vi "Data Transmission DAO.vi"(7 "refnum":T1, 8 "error in (no error)":errorcluster, 9 "Port Number In":u16, 10 "Wait For Notification Timeout In":i32=1000, 11 "Persistent DAO Actions":T2) -> (0 "error out":errorcluster, 1 "Port Number Out":u16, 2 "Wait For Notification Timeout Out":i32=1000, 3 "Notification Name Out":string="DataAvailableForTransmission", 4 "refnum out":T1)   [LabVIEW 2009]
uses:
  Metadata/Persistant DAO Actions.ctl
  <vilib>/Utility/config.llb/Config Data RefNum.ctl
  <vilib>/Utility/config.llb/Read Key (String).vi
  <vilib>/Utility/config.llb/Read Key (I32).vi
  <vilib>/Utility/config.llb/Read Key (U32).vi
  <vilib>/Utility/config.llb/Write Key (String).vi
  <vilib>/Utility/config.llb/Write Key (I32).vi
  <vilib>/Utility/config.llb/Write Key (U32).vi
  <vilib>/Utility/config.llb/NI_LVConfig.lvlib
panel:
  in  "Notification Name In":string="DataAvailableForTransmission"
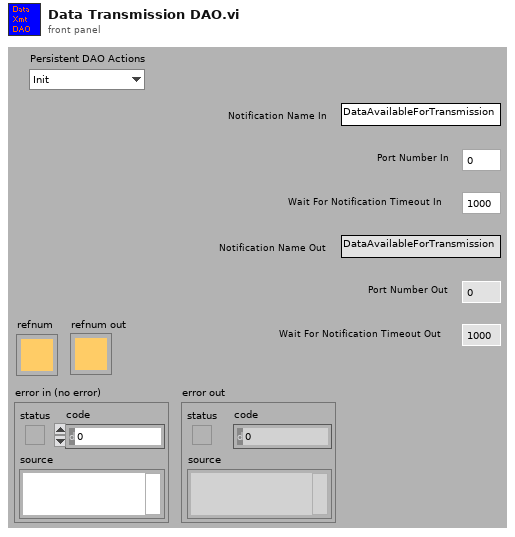
[diagram p1: front panel]
types:
  T1 = typedef "NI_LVConfig.lvlib/Config Data RefNum.ctl" = refnum<k1>
  T2 = typedef "Persistant DAO Actions.ctl" = enum16{"Init", "Get", "Set", "Load", "Save"}
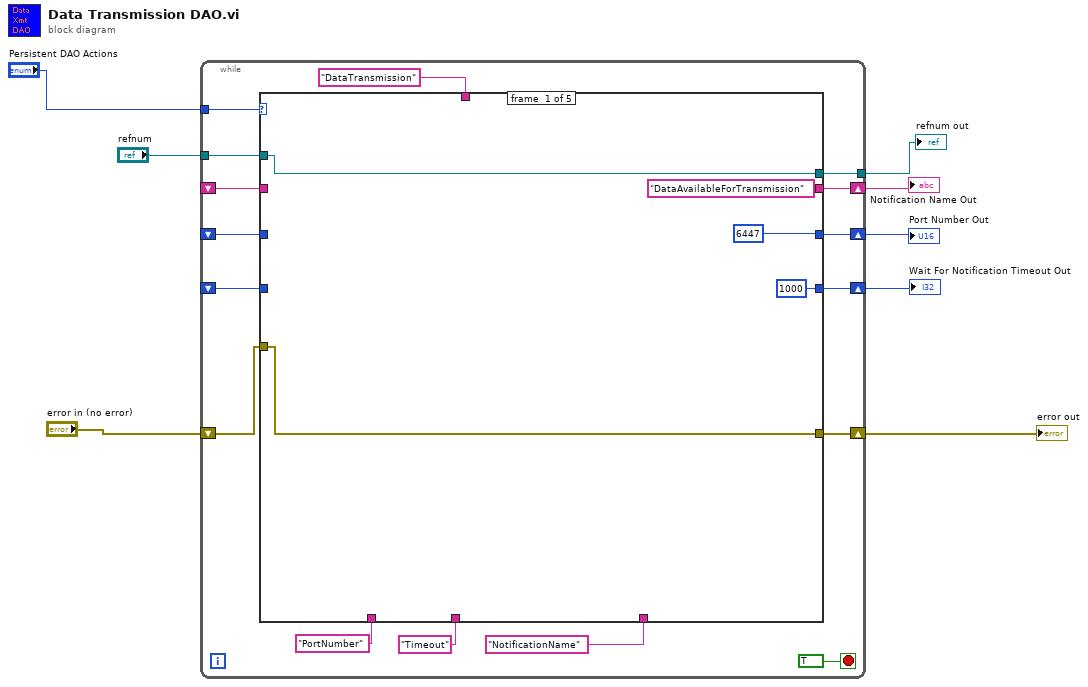
[diagram p0: block diagram]
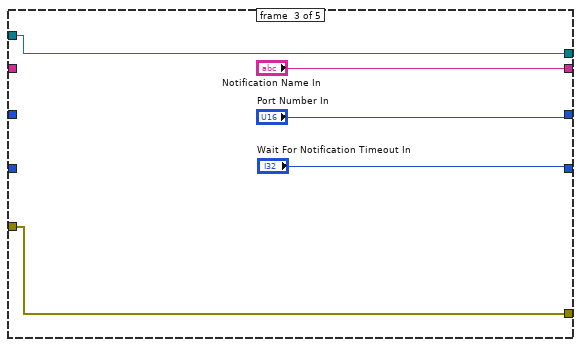
[diagram p3: hidden frame]
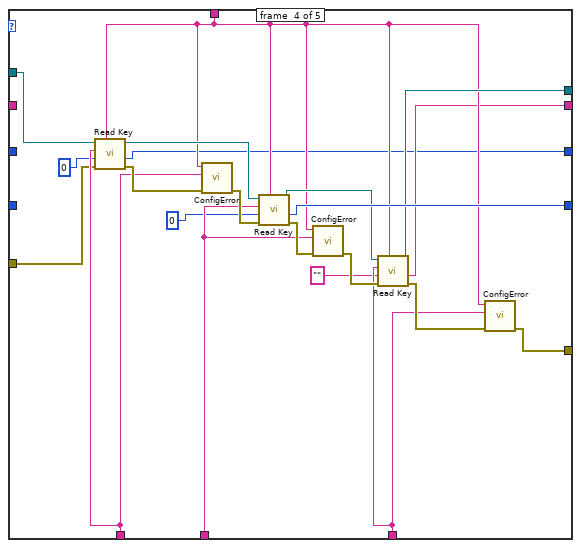
[diagram p4: hidden frame]
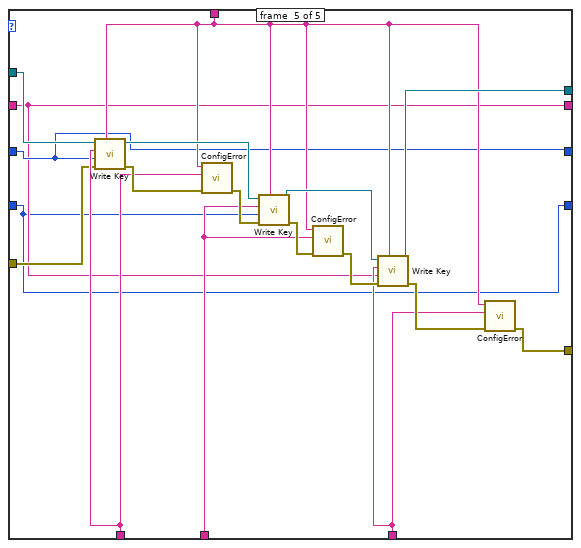
[diagram p5: hidden frame]
diagram:
  n1 = while {
    tunnel: "Persistent DAO Actions" -> [w23]
    shift-right: [w22] -> w7
    shift-left: _ -> [w20]
    shift-right: [w21] -> w6
    shift-left: _ -> [w19]
    shift-right: [w18] -> w5
    shift-left: _ -> [w17]
    tunnel: "refnum" -> [w14]
    shift-right: [w11] -> w2
    shift-left: "error in (no error)" -> [w12]
    tunnel: [w10] -> w1
    stop <- TRUE stop-if-true
    n2 = case shown="\"Save\"" w23 {
      tunnel: ["DataAvailableForTransmission" ("Notification Name In") w34 "Notification Name In" w43 w62] -> w22
      tunnel: [u16 6447 ("Port Number In") w30 "Port Number In" w41 w63] -> w21
      tunnel: w20 -> [_ w34 _ _ w62]
      tunnel: w19 -> [_ w30 _ _ w63]
      tunnel: [1000 ("Wait For Notification Timeout In") w33 "Wait For Notification Timeout In" w52 w61] -> w18
      tunnel: w17 -> [_ w33 _ _ w61]
      tunnel: "DataTransmission" -> [_ _ _ w46 w66]
      tunnel: "PortNumber" -> [_ _ _ w59 w77]
      tunnel: w14 -> [w27 w31 w36 w58 w76]
      tunnel: "Timeout" -> [_ _ _ w54 w72]
      tunnel: w12 -> [w26 w32 w37 w51 w71]
      tunnel: [w26 w32 w37 w42 w64] -> w11
      tunnel: [w27 w31 w36 w47 w67] -> w10
      tunnel: "NotificationName" -> [_ _ _ w45 w65]
      frame #0 {
      }
      frame #1 {
      }
      frame #2 {
      }
      frame #3 {
        n3 = call-poly <vilib>:"Read Key.vi"("section"=w46, "error in (no error)"=w51, "default value"=u16 0 ("Port Number In"), "key"=w59, "refnum"=w58) -> ("error out"=w60:errorcluster, "value"=w41:u32, "refnum out"=w55:T1)  [unwired: 4 out]
        n4 = call "ConfigError.vi"("error in (no error)"=w60, "Key"=w59, "Section"=w46) -> ("error out"=w56:errorcluster)  [unwired: 8 out]
        n5 = call-poly <vilib>:"Read Key.vi"("section"=w46, "error in (no error)"=w56, "default value"=0 ("Wait For Notification Timeout In"), "key"=w54, "refnum"=w55) -> ("error out"=w57:errorcluster, "value"=w52:i32, "refnum out"=w48:T1)  [unwired: 4 out]
        n6 = call "ConfigError.vi"("error in (no error)"=w57, "Key"=w54, "Section"=w46) -> ("error out"=w49:errorcluster)  [unwired: 8 out]
        n7 = call-poly <vilib>:"Read Key.vi"("section"=w46, "error in (no error)"=w49, "default value"="", "key"=w45, "refnum"=w48) -> ("error out"=w50:errorcluster, "value"=w43:string, "refnum out"=w47:T1)  [unwired: 1 in, 3 out]
        n8 = call "ConfigError.vi"("error in (no error)"=w50, "Key"=w45, "Section"=w46) -> ("error out"=w42:errorcluster)  [unwired: 8 out]
      }
      frame #4 {
        n9 = call-poly <vilib>:"Write Key.vi"("section"=w66, "error in (no error)"=w71, "value"=w63, "key"=w77, "refnum"=w76) -> ("error out"=w78:errorcluster, "refnum out"=w73:T1)  [unwired: 5 out]
        n10 = call "ConfigError.vi"("error in (no error)"=w78, "Key"=w77, "Section"=w66) -> ("error out"=w74:errorcluster)  [unwired: 8 out]
        n11 = call-poly <vilib>:"Write Key.vi"("section"=w66, "error in (no error)"=w74, "value"=w61, "key"=w72, "refnum"=w73) -> ("error out"=w75:errorcluster, "refnum out"=w68:T1)  [unwired: 5 out]
        n12 = call "ConfigError.vi"("error in (no error)"=w75, "Key"=w72, "Section"=w66) -> ("error out"=w69:errorcluster)  [unwired: 8 out]
        n13 = call-poly <vilib>:"Write Key.vi"("section"=w66, "error in (no error)"=w69, "value"=w62, "key"=w65, "refnum"=w68) -> ("error out"=w70:errorcluster, "refnum out"=w67:T1)  [unwired: 1 in, 4 out]
        n14 = call "ConfigError.vi"("error in (no error)"=w70, "Key"=w65, "Section"=w66) -> ("error out"=w64:errorcluster)  [unwired: 8 out]
      }
    }
  }
  "Port Number Out" <- w6
  "Notification Name Out" <- w7
  "error out" <- w2
  "Wait For Notification Timeout Out" <- w5
  "refnum out" <- w1
